vi "StrictFollower Setter.vi"(0 "DeviceReference":T1, 3 "Update Frequency (Hz)":dbl=100.0, 5 "MasterID":i32) -> (4 "DeviceReference Out":T1)   [LabVIEW 2020]
doc: "Follow the motor output of another Talon while ignoring the master's invert setting.\nIf Talon is in torque control, the torque is copied - which will increase the total torque applied. If Talon is in percent supply output control, the duty cycle is matched. Motor direction is strictly determined by the configured invert and not the master. If you want motor direction to match or oppose the master, use FollowerRequest instead."
uses:
  DeviceReference.ctl
  <userlib>/CTRE_PhoenixTools/CTRE_PhoenixTools.lvlib
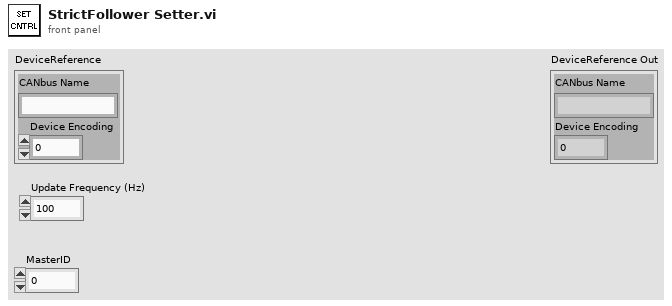
[diagram p1: front panel]
types:
  T1 = typedef "DeviceReference.ctl" = cluster{"CANbus Name":string, "Device Encoding":u32}
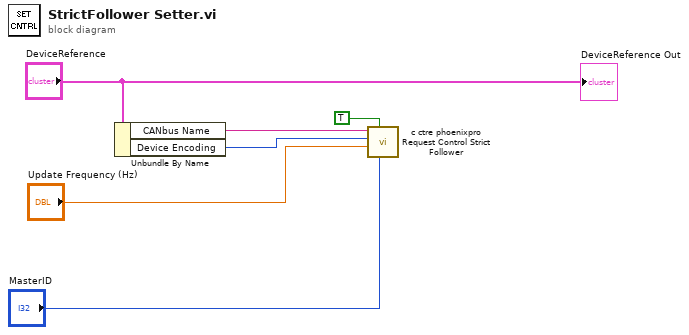
[diagram p0: block diagram]
diagram:
  n1 = Unbundle By Name("DeviceReference") -> ("CANbus Name"=w5:string, "Device Encoding"=w4:u32)
  n2 = call <userlib>:"c ctre phoenixpro Request Control Strict Follower.vi"("MasterID"="MasterID", "cancelOtherRequests"=TRUE, "updateTime"="Update Frequency (Hz)", "ecuEncoding"=w4, "canbus"=w5) -> ()  [unwired: 5 in, 2 out]
  "DeviceReference Out" <- "DeviceReference"
